vi "CloseHardware.vi"(8 "error in (no error)":errorcluster, 11 "NewportXPS in":refnum<class "NewportXPS.lvclass">) -> (0 "error out":errorcluster)   [LabVIEW 2020, in "NewportXPS.lvclass"]
uses:
  NewportXPS.lvclass
  NewportXPS.lvclass/NewportXPS.ctl
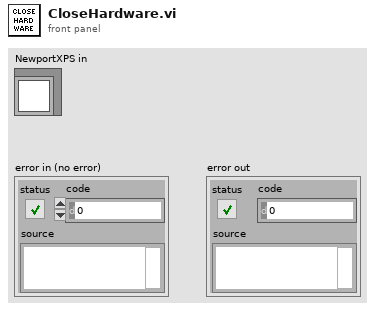
[diagram p1: front panel]
types:
  T1 = cluster{"connection TCP":refnum<k5>, "LogTo File":bool, "Log File refnum":refnum<file>, "no error if error log":bool}
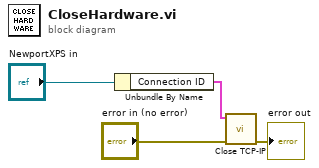
[diagram p0: block diagram]
diagram:
  n1 = Unbundle By Name("NewportXPS in") -> ("Connection ID"=w4:T1)
  n2 = call "Close TCP-IP.vi"("error in (no error)"="error in (no error)", "connection ID in"=w4) -> ("Error out"=→"error out":errorcluster)  [unwired: 9 in]
